vi "Axsun Control VDL.vi"(8 "error in (no error)":errorcluster) -> (0 "error in (no error) 2":errorcluster)   [LabVIEW 2015, in "Axsun_1310_SS.lvclass"]
uses:
  Axsun_1310_SS.lvclass
  C:/Program Files (x86)/Axsun/Axsun OCT Control/AxsunOCTControl.dll
  Axsun VDL Global.vi
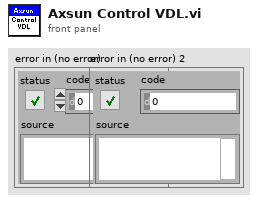
[diagram p1: front panel]
types:
  T1 = typedef "Axsun_1310_SS.lvclass/Axsun VDL Typedef.ctl" = cluster{"Speed (mm/s)":dbl, "Position (mm)":dbl, "Home":bool}
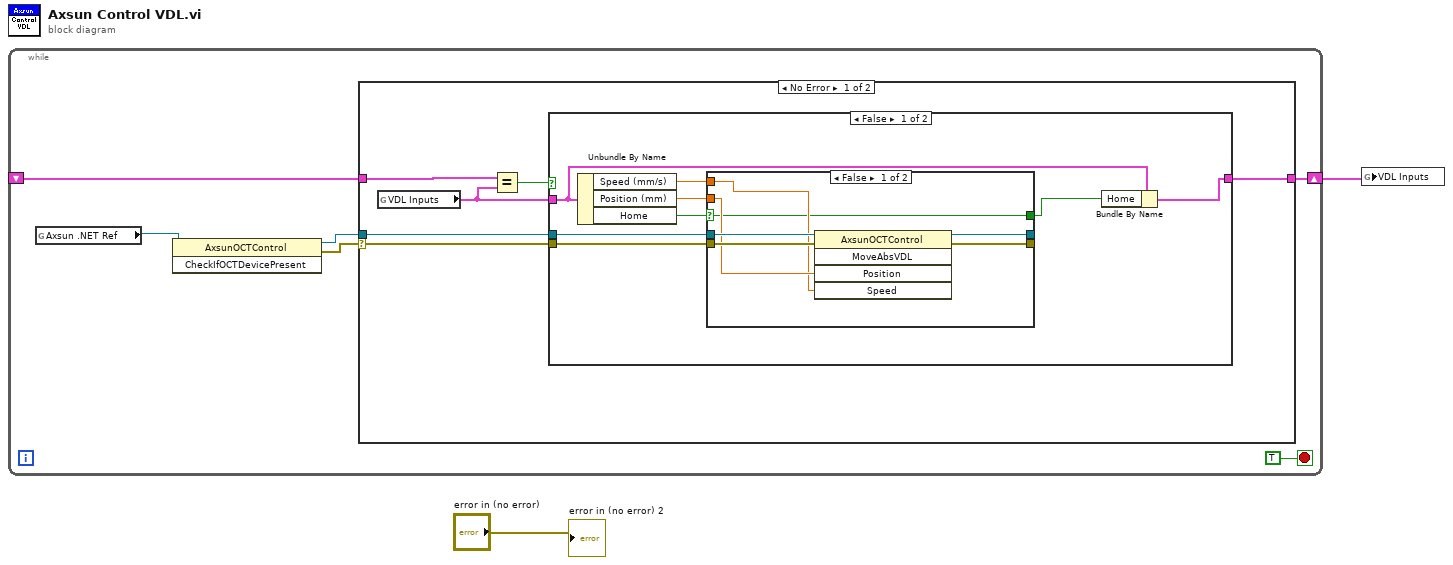
[diagram p0: block diagram]
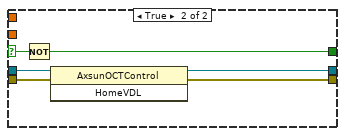
[diagram p2: hidden frame]
diagram:
  n1 = while {
    shift-right: [w7] -> w1
    shift-left: _ -> [w5]
    stop <- TRUE stop-if-true
    n2 = global read "Axsun VDL Global.vi" "Axsun .NET Ref"() -> (w6:refnum<k24>)
    n3 = invoke class="AxsunOCTControl" method="CheckIfOCTDevicePresent"(reference=w6) -> (reference out=w4:refnum<k24>, error out=w3:errorcluster)  [unwired: 2 in, 1 out]
    n4 = case shown="No Error" w3 {
      selector: w3 -> [w9 _]
      tunnel: [w11 w37] -> w7
      tunnel: w5 -> [w14 w37]
      tunnel: w4 -> [w10 _]
      frame No Error {
        n5 = global read "Axsun VDL Global.vi" "VDL Inputs"() -> (w12:T1)
        n6 = Equal?(x=w14, y=w12) -> (x = y?=w13:bool)
        n7 = case shown="False" w13 {
          tunnel: w12 -> [w19 w36]
          tunnel: [w18 w36] -> w11
          tunnel: w10 -> [w22 _]
          tunnel: w9 -> [w21 _]
          frame False {
            n8 = Unbundle By Name(w19) -> ("Speed (mm/s)"=w16:dbl, "Position (mm)"=w15:dbl, "Home"=w20:bool)
            n9 = case shown="False" w20 {
              selector: w20 -> [w23 w31]
              tunnel: w22 -> [w29 w35]
              tunnel: w21 -> [w28 w34]
              tunnel: [w26 w33] -> _
              tunnel: [w27 w32] -> _
              tunnel: [w23 w30] -> w17
              tunnel: w16 -> [w24 _]
              tunnel: w15 -> [w25 _]
              frame False {
                n10 = invoke class="AxsunOCTControl" method="MoveAbsVDL"(reference=w29, error in=w28, "Position"=w25, "Speed"=w24) -> (reference out=w27:refnum<k24>, error out=w26:errorcluster)  [unwired: 1 in, 3 out]
              }
              frame True {
                n11 = Not(x=w31) -> (.not. x?=w30:bool)
                n12 = invoke class="AxsunOCTControl" method="HomeVDL"(reference=w35, error in=w34) -> (reference out=w32:refnum<k24>, error out=w33:errorcluster)  [unwired: 1 in, 1 out]
              }
            }
            n13 = Bundle By Name(cluster=w19, "Home"=w17) -> (w18:T1)
          }
          frame True {
            # "do nothing"
          }
        }
      }
      frame Error {
      }
    }
  }
  n14 = global write "Axsun VDL Global.vi" "VDL Inputs"(w1) -> ()
  "error in (no error) 2" <- "error in (no error)"
